vi "Reset ABS Enc.vi"(8 "error in (no error)":errorcluster, 11 "SGDV_Ctrl_Class in":refnum<class "SGDV_Ctrl_Class.lvclass">) -> (0 "error out":errorcluster, 2 "Init Motor Data":T1, 3 "SGDV_Ctrl_Class out":refnum<class "SGDV_Ctrl_Class.lvclass">)   [LabVIEW 2013, in "SGDV_Ctrl_v13_lib.lvlib" / "SGDV_Ctrl_Class.lvclass"]
uses:
  SGDV_Ctrl_Class.lvclass
  Controls and General VIs/Init Motor Data.ctl
  SGDV_Ctrl_Class.lvclass/SGDV_Ctrl_Class.ctl
  SGDV_Ctrl_v13_lib.lvlib
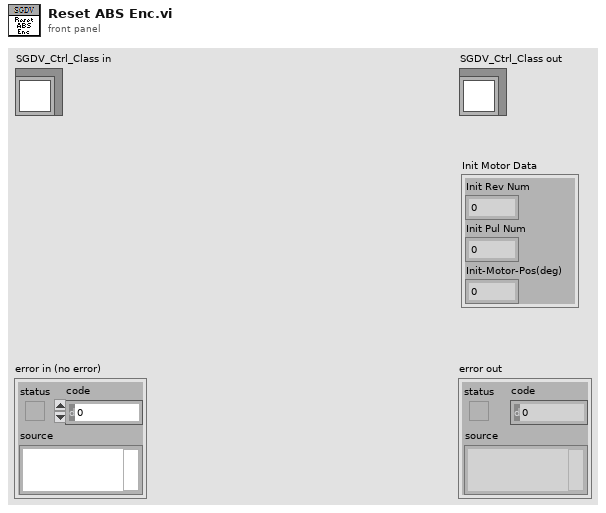
[diagram p1: front panel]
types:
  T1 = typedef "SGDV_Ctrl_v13_lib.lvlib/Init Motor Data.ctl" = cluster{"Init Rev Num":i32, "Init Pul Num":i32, "Init-Motor-Pos(deg)":dbl}
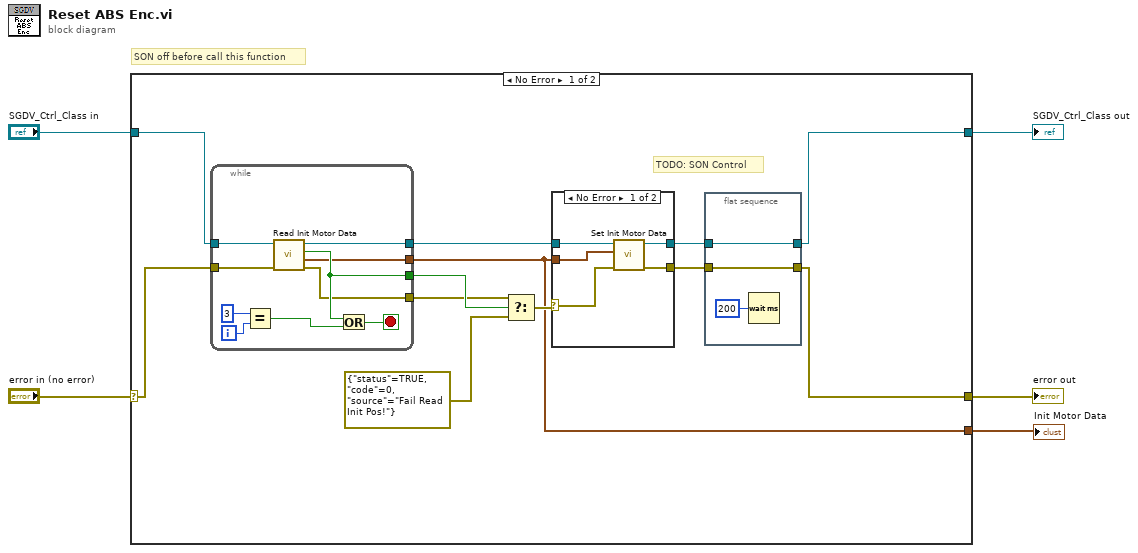
[diagram p0: block diagram]
diagram:
  # "SON off before call this function"
  n1 = case shown="No Error" "error in (no error)" {
    selector: "error in (no error)" -> [w9 w39]
    tunnel: [w8 w39] -> w4
    tunnel: [w7 w38] -> w2
    tunnel: "SGDV_Ctrl_Class in" -> [w10 w38]
    tunnel: [w6 _] -> w1
    frame No Error {
      # "TODO: SON Control"
      n2 = while {
        tunnel: [w33] -> w13
        tunnel: [w32] -> w17
        tunnel: w10 -> [w31]
        tunnel: w9 -> [w30]
        tunnel: [w29] -> w6
        tunnel: [w28] -> w16
        i -> [w37]
        stop <- w34 stop-if-true
        n3 = Equal?(x=3, y=w37) -> (x = y?=w35:bool)
        n4 = call "Read Init Motor Data.vi"("error in (no error)"=w30, "SGDV_Ctrl_Class in"=w31) -> ("error out"=w28:errorcluster, "Init Motor Data"=w29:T1, "Get Serial Data?"=w32:bool, "SGDV_Ctrl_Class out"=w33:refnum<class "SGDV_Ctrl_Class.lvclass">)  [unwired: 6 in]
        n5 = Or(x=w32, y=w35) -> (x .or. y?=w34:bool)
      }
      n6 = Select(t=w16, s=w17, f=errorcluster {"status"=TRUE, "code"=0, "source"="Fail Read Init Pos!"}) -> (s? t:f=w14:errorcluster)
      n7 = case shown="No Error" w14 {
        selector: w14 -> [w23 w26]
        tunnel: w13 -> [w25 w27]
        tunnel: w6 -> [w24 _]
        tunnel: [w22 w27] -> w12
        tunnel: [w21 w26] -> w11
        frame No Error {
          n8 = call "Set Init Motor Data.vi"("error in (no error)"=w23, "Init Motor Data"=w24, "SGDV_Ctrl_Class in"=w25) -> ("error out"=w21:errorcluster, "SGDV_Ctrl_Class out"=w22:refnum<class "SGDV_Ctrl_Class.lvclass">)  [unwired: 7 in]
        }
        frame Error {
        }
      }
      n9 = flat-sequence {
        tunnel: w12 -> [w20]
        tunnel: [w20] -> w7
        tunnel: w11 -> [w19]
        tunnel: [w19] -> w8
        frame #0 {
          n10 = Wait (ms)(milliseconds to wait=u32 200) -> ()  [unwired: 1 out]
        }
      }
    }
    frame Error {
    }
  }
  "error out" <- w4
  "SGDV_Ctrl_Class out" <- w2
  "Init Motor Data" <- w1
